vi "Pump Configure.vi"(8 "error in (no error)":errorcluster, 10 "Message Data":variant, 11 "Data Cluster":T1 {"Pump Info"."Direction" items=["CW", "CCW"]; "Pump Info"."Speed" format="%03.0f"}) -> (0 "error out":errorcluster, 2 "Send Resp":bool, 3 "Data Cluster out":T1 {"Pump Info"."Direction" items=["CW", "CCW"]; "Pump Info"."Speed" format="%03.0f"})   [LabVIEW 2020, in "Pump.lvlib"]
uses:
  Pump.lvlib
  Pump Hardware Configuration.ctl
  support/Message Queue/Message Cluster.ctl
  support/Message Queue/Message Queue.lvlib
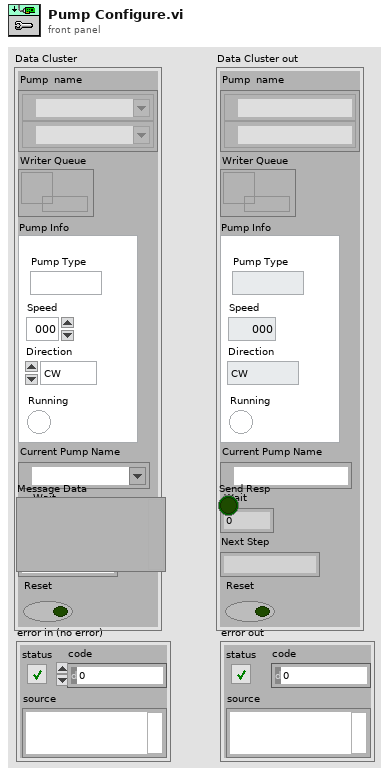
[diagram p1: front panel]
types:
  T1 = typedef "Pump.lvlib/Pump Hardware Configuration.ctl" = cluster{"Pump  name":refnum<visa-resource-name>[], "Writer Queue":refnum<queue>, "Pump Info":cluster{"Pump Type":string, "Speed":i32, "Direction":u16, "Running":bool}, "Current Pump Name":refnum<visa-resource-name>, "Wait":dbl, "Next Step":string, "Reset":bool}
  T2 = typedef "Message Queue.lvlib/Message Cluster.ctl" = cluster{"Message":string, "Message Data":variant}
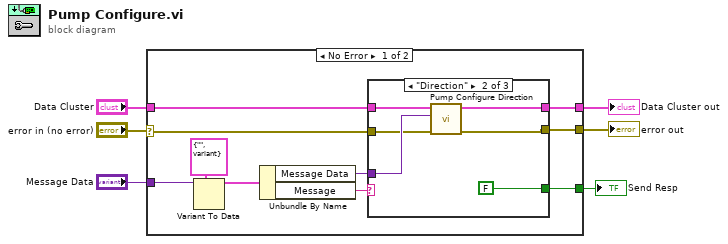
[diagram p0: block diagram]
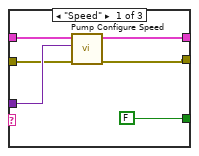
[diagram p2: hidden frame]
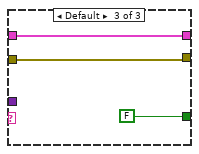
[diagram p3: hidden frame]
diagram:
  n1 = case shown="No Error" "error in (no error)" {
    selector: "error in (no error)" -> [w9 w32]
    tunnel: [w16 w32] -> w6
    tunnel: "Data Cluster" -> [w15 w33]
    tunnel: [w14 w33] -> w4
    tunnel: "Message Data" -> [w10 _]
    tunnel: [w7 _] -> w1
    frame No Error {
      n2 = Variant To Data(type=T2 {"Message"="", "Message Data"=variant} ("element"), Variant=w10) -> (data=w12:T2)  [unwired: 1 in, 1 out]
      n3 = Unbundle By Name(w12) -> ("Message Data"=w8:variant, "Message"=w13:string)
      n4 = case shown="\"Direction\"" w13 {
        tunnel: w8 -> [w19 w25 _]
        tunnel: [w20 w26 w30] -> w14
        tunnel: w15 -> [w21 w27 w30]
        tunnel: w9 -> [w18 w24 w29]
        tunnel: [w17 w23 w29] -> w16
        tunnel: [FALSE ("Send Resp") FALSE ("Send Resp") FALSE ("Send Resp")] -> w7
        frame "Speed" {
          n5 = call "Pump Configure Speed.vi"("error in (no error)"=w18, "Message Data"=w19, "Data Cluster in"=w21) -> ("error out"=w17:errorcluster, "Data Cluster out"=w20:T1)  [unwired: 7 in]
        }
        frame "Direction" {
          n6 = call "Pump Configure Direction.vi"("error in (no error)"=w24, "Message Data"=w25, "Data Cluster in"=w27) -> ("error out"=w23:errorcluster, "Data Cluster out"=w26:T1)  [unwired: 7 in]
        }
        frame Default {
        }
      }
    }
    frame Error {
    }
  }
  "error out" <- w6
  "Data Cluster out" <- w4
  "Send Resp" <- w1
